vi "Pre-Process.vi"(11 "Element in":refnum<class "Element.lvclass">) -> (3 "Element out":refnum<class "Element.lvclass">)   [LabVIEW 2021, in "Element.lvclass"]
uses:
  Element.lvclass
  Element.lvclass/Element.ctl
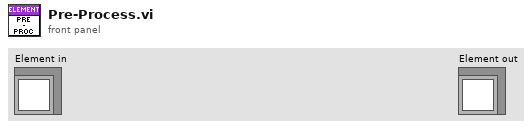
[diagram p1: front panel]
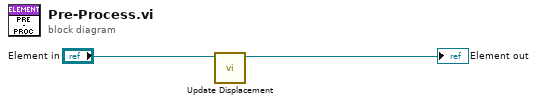
[diagram p0: block diagram]
diagram:
  n1 = call "Update Displacement.vi"("Element in"="Element in") -> ("Element out"=→"Element out":refnum<class "Element.lvclass">)  [unwired: 10 in]
